vi "Get Data Notifier.vi"(6 "Data Notifier Name":string, 7 "Task Name":string, 8 "error in (no error)":errorcluster, 11 "Series Base in":refnum<class "Series Base.lvclass">) -> (0 "error out":errorcluster, 2 "Data Notifier":refnum<notifier>, 3 "Series Base out":refnum<class "Series Base.lvclass">)   [LabVIEW 2023, in "HAL GOOP4.lvlib" / "Series Base.lvclass"]
uses:
  Series Base.lvclass
  Series Base.lvclass/Series Base.ctl
  Task/Task Base/Task Base.lvclass/Task Base.ctl
  <vilib>/Utility/error.llb/Error Cluster From Error Code.vi
  Task/Task Base/Task Base.lvclass
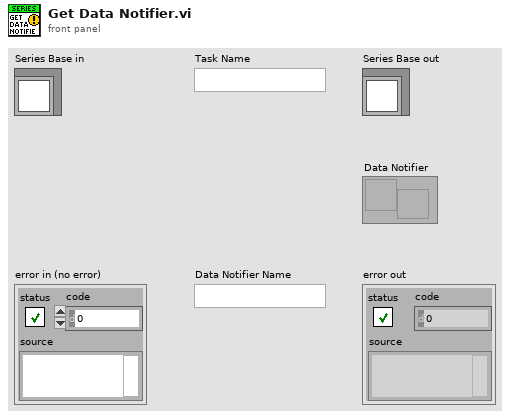
[diagram p1: front panel]
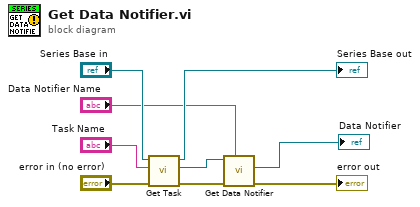
[diagram p0: block diagram]
diagram:
  n1 = call "Get Task.vi"("error in (no error)"="error in (no error)", "Task Name"="Task Name", "Series Base in"="Series Base in") -> ("error out"=w4:errorcluster, "Task"=w3:refnum<class "Task Base.lvclass">, "Series Base out"=→"Series Base out":refnum<class "Series Base.lvclass">)  [unwired: 6 in]
  n2 = call "Get Data Notifier.vi"("Target Name"="Data Notifier Name", "error in (no error)"=w4, "Task Base in"=w3) -> ("error out"=→"error out":errorcluster, "Data Notifier"=→"Data Notifier":refnum<notifier>)  [unwired: 6 in, 1 out]
